vi "Utility Log to File.vi"(8 "error in (no error)":errorcluster, 9 "Additional Notes":string, 10 "Command":string, 11 "Log File Path":path) -> (0 "error out":errorcluster)   [LabVIEW 2020, in "ChromTech Series I Drivers.lvlib"]
doc: "Logs a given command to the specified logging file. A timestamp of the current time is logged with the command, along with any error codes present in the \"error in\" parameter. The \"error out\" return value only returns errors from the logging itself; errors present in the \"error in\" parameter are ignored and used for logging purposes only."
uses:
  <instrlib>/RxnRover/ChromtechSeriesIDriver/ChromTech Series I Drivers.lvlib
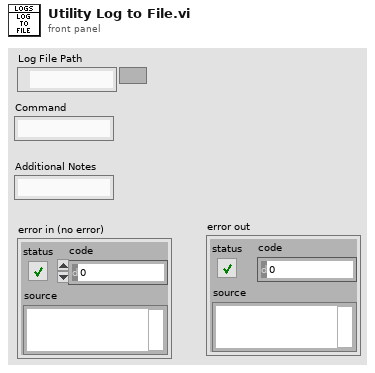
[diagram p1: front panel]
types:
  T1 = enum16{"open", "replace", "create", "open or create", "replace or create", "replace or create with confirmation"}
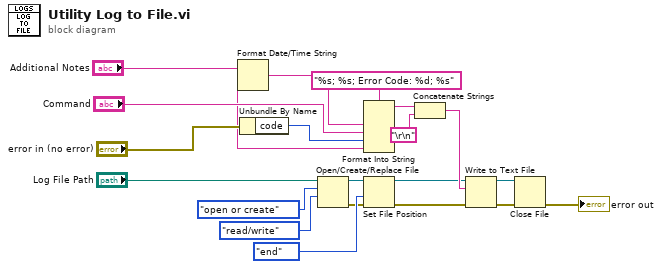
[diagram p0: block diagram]
diagram:
  n1 = Format Date/Time String() -> (date/time string=w2:string)  [unwired: 3 in]
  n2 = Unbundle By Name("error in (no error)") -> ("code"=w18:i32)
  n3 = Open/Create/Replace File(file path (use dialog)="Log File Path", operation (0:open)=T1."open or create", access (0:read/write)=enum16{"read/write", "read-only", "write-only"}."read/write") -> (refnum out=w6:refnum<file>, error out=w5:errorcluster)  [unwired: 3 in, 1 out]
  n4 = Format Into String(format string="%s; %s; Error Code: %d; %s", w2, "Command", w18, "Additional Notes") -> (resulting string=w15:string)  [unwired: 2 in, 1 out]
  n5 = Set File Position(refnum=w6, from (0:start)=enum16{"start", "end", "current"}."end", error in=w5) -> (refnum out=w8:refnum<file>, error out=w7:errorcluster)  [unwired: 1 in]
  n6 = Concatenate Strings(w15, "\r\n") -> (w16:string)
  n7 = Write to Text File(file (use dialog)=w8, text=w16, error in=w7) -> (refnum out=w10:refnum<file>, error out=w9:errorcluster)  [unwired: 1 in, 1 out]
  n8 = Close File(refnum=w10, error in=w9) -> (error out=→"error out":errorcluster)  [unwired: 1 out]
